vi "Write 2D Compass Phase Scale.vi"(8 "error in (no error)":errorcluster, 10 "Phase Scale":bool=TRUE, 11 "2D Compass.lvclass in":refnum<class "2D Compass.lvclass">) -> (0 "error out":errorcluster, 3 "2D Compass.lvclass out":refnum<class "2D Compass.lvclass">)   [LabVIEW 2020, in "2D Compass.lvclass"]
uses:
  <vilib>/Math Plots/2D Math Plots/2D Compass/2D Compass/2D Compass.lvclass
  <vilib>/Math Plots/2D Math Plots/2D Compass/2D Compass/2D Compass.lvclass/2D Compass.ctl
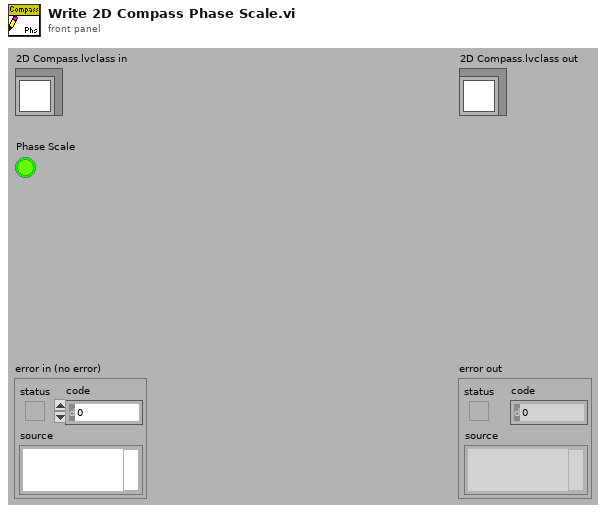
[diagram p1: front panel]
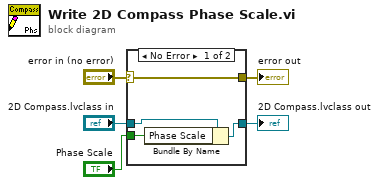
[diagram p0: block diagram]
diagram:
  n1 = case shown="No Error" "error in (no error)" {
    selector: "error in (no error)" -> [w9 w10]
    tunnel: [w9 w10] -> w4
    tunnel: [w7 w11] -> w2
    tunnel: "2D Compass.lvclass in" -> [w8 w11]
    tunnel: "Phase Scale" -> [w6 _]
    frame No Error {
      n2 = Bundle By Name(cluster=w8, "Phase Scale"=w6) -> (w7:refnum<class "2D Compass.lvclass">)
    }
    frame Error {
    }
  }
  "error out" <- w4
  "2D Compass.lvclass out" <- w2
